vi "Main UI.vi"() -> ()   [LabVIEW 2017]
panel:
  in  "Close":bool
  in  "Help":bool
  in  "Measurement Tree":string(tree)
  in  "Add":bool
  in  "Remove":bool
  in  "Tune":bool
  in  "Stop":bool
  in  "Play":bool
  in  "Parameters Tab Control":T1(tab)
  in  "Accumulation":dbl caption="Numeric"
  in  "Delay Time":dbl[unit]
  in  "Integration Time":dbl[unit]
  in  "Scan Resolution":dbl[unit]
  in  "Number of Points":dbl caption="Numeric"
  in  "Stop Wavelength":dbl[unit]
  in  "Start Wavelength":dbl[unit]
  in  "Sync":bool
  in  "Save":bool
  out "Signal Intensity Monitor":cluster{"X":dbl, "Y":dbl}[](graph) caption="XY Graph"
  out "Intensity":cluster{"X":dbl, "Y":dbl}[](graph) caption="XY Graph"
  in  "Graph Line Chart":bool
  in  "Cloud Download":bool
  in  "Camera":bool
  in  "Save Settings":bool
  in  "Print":bool
  out "Status":string="Program Status"
  out "Progress":u8(slide)=45 scale=0.0..100.0
  # "Laser Measurement Tool v.0.1"
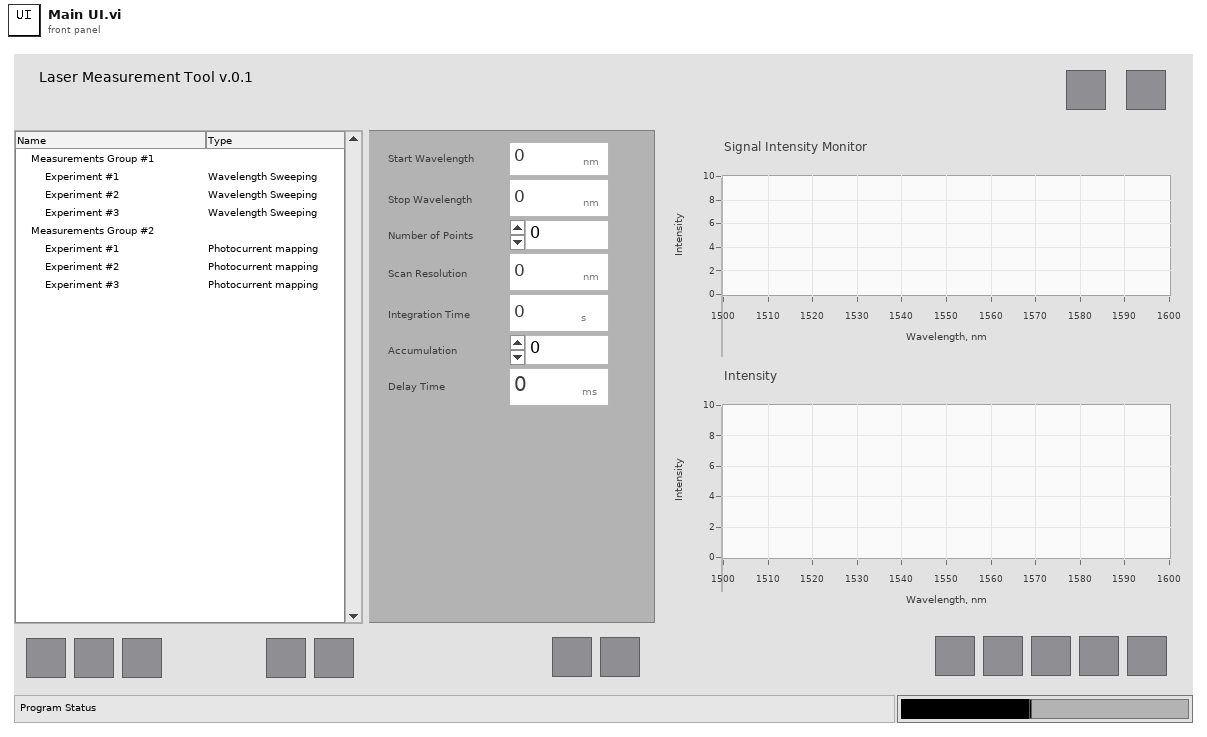
[diagram p1: front panel]
types:
  T1 = enum32{"Wavelength Sweeping", "Photocurrent mapping"}
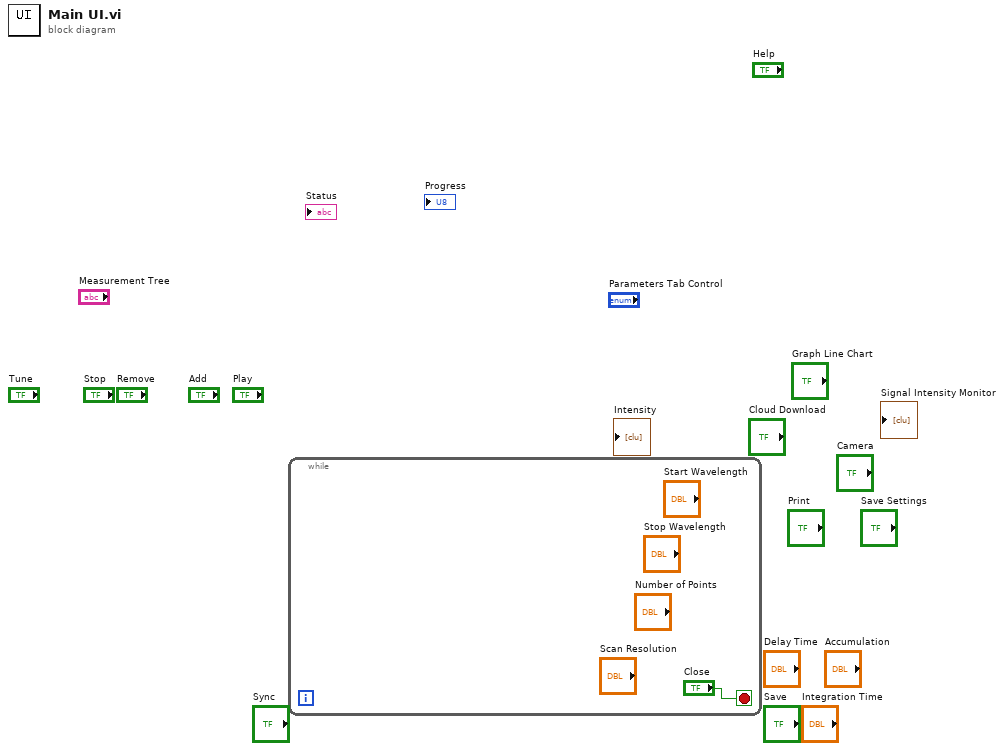
[diagram p0: block diagram]
diagram:
  n1 = while {
    stop <- "Close" stop-if-true
  }
